vi "Configure External Sweep.vi"(8 "error in (no error)":errorcluster, 9 "Stop Method (0: ssStopWithinTol)":i32(ring) items=["ssStopWithinTol", "ssStopOnReturn"], 10 "Start Method (0: ssStartWithinTol)":i32(ring) items=["ssStartWithinTol", "ssStartWithinRange", "ssStartAnywhere"], 11 "VISA resource name":refnum<visa-resource-name>) -> (0 "error out":errorcluster, 3 "VISA resource name out":refnum<visa-resource-name>)   [LabVIEW 2014, in "Stanford Research SR1.lvlib"]
doc: "Configures the attributes for the External Sweep."
uses:
  Stanford Research SR1.lvlib
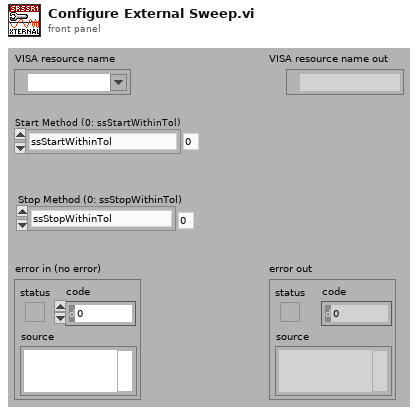
[diagram p1: front panel]
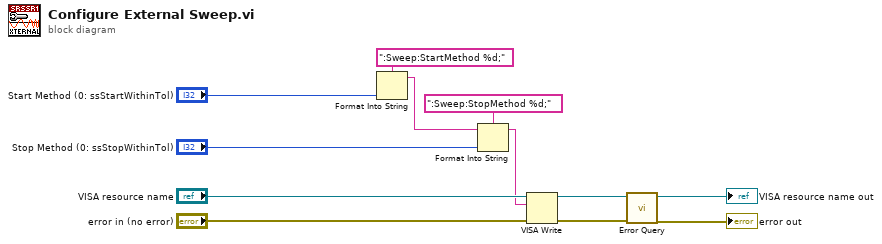
[diagram p0: block diagram]
diagram:
  n1 = Format Into String(format string=":Sweep:StartMethod %d;", "Start Method (0: ssStartWithinTol)") -> (resulting string=w2:string)  [unwired: 2 in, 1 out]
  n2 = Format Into String(format string=":Sweep:StopMethod %d;", initial string=w2, "Stop Method (0: ssStopWithinTol)") -> (resulting string=w1:string)  [unwired: 1 in, 1 out]
  n3 = VISA Write(VISA resource name="VISA resource name", write buffer=w1, error in (no error)="error in (no error)") -> (VISA resource name out=w8:refnum<visa-resource-name>, error out=w7:errorcluster)  [unwired: 1 out]
  n4 = call "Error Query.vi"("error in (no error)"=w7, "VISA resource name"=w8) -> ("error out"=→"error out":errorcluster, "VISA resource name out"=→"VISA resource name out":refnum<visa-resource-name>)  [unwired: 6 in, 2 out]
